vi "sv_Get Level Detector Type String.vi"(4 "level detector type":T1=19 items=["Value"=19, "DC"=11, "AC"=12, "RMS^2"=13, "RMS"=14, "Peak"=15, "Peak to peak"=16, "Unknown"=99]) -> (1 "level detector type string":string)   [LabVIEW 2017]
uses:
  <vilib>/addons/_NISVFA/_Shared subVIs/Controls/NI Level Detector Type.ctl
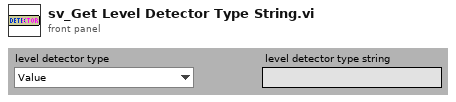
[diagram p1: front panel]
types:
  T1 = typedef "NI Level Detector Type.ctl" = i32
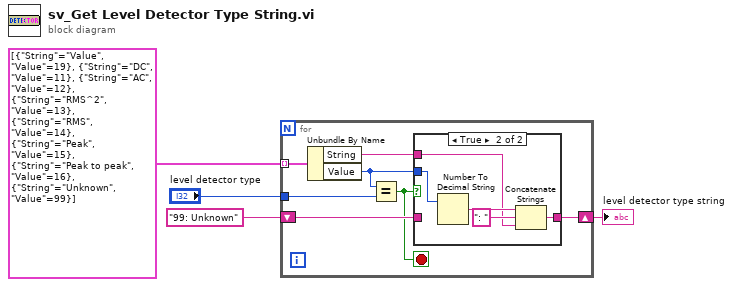
[diagram p0: block diagram]
diagram:
  n1 = for {
    tunnel: cluster{"String":string, "Value":i32}[] [{"String"="Value", "Value"=19}, {"String"="DC", "Value"=11}, {"String"="AC", "Value"=12}, {"String"="RMS^2", "Value"=13}, {"String"="RMS", "Value"=14}, {"String"="Peak", "Value"=15}, {"String"="Peak to peak", "Value"=16}, {"String"="Unknown", "Value"=99}] ("Strings And Values []") -> [w11] mode=indexing
    shift-right: [w8] -> w2
    shift-left: "99: Unknown" ("String") -> [w6]
    tunnel: "level detector type" -> [w10]
    stop <- w5 stop-if-true
    n2 = Unbundle By Name(w11) -> ("String"=w9:string, "Value"=w7:i32)
    n3 = Equal?(x=w7, y=w10) -> (x = y?=w5:bool)
    n4 = case shown="True" w5 {
      tunnel: w9 -> [_ w15]
      tunnel: [w12 w14] -> w8
      tunnel: w7 -> [_ w13]
      tunnel: w6 -> [w12 _]
      frame False {
      }
      frame True {
        n5 = Number To Decimal String(number=w13) -> (decimal integer string=w16:string)  [unwired: 1 in]
        n6 = Concatenate Strings(w16, ": " ("string"), w15) -> (w14:string)
      }
    }
  }
  "level detector type string" <- w2
